vi "魔法攻击.vi"() -> ()   [LabVIEW 2018]
panel:
  out "滑动杆":dbl(slide) scale=0.0..10.0
  out "布尔 2":bool
  out "布尔":bool
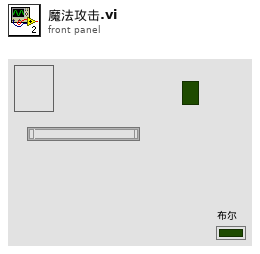
[diagram p1: front panel]
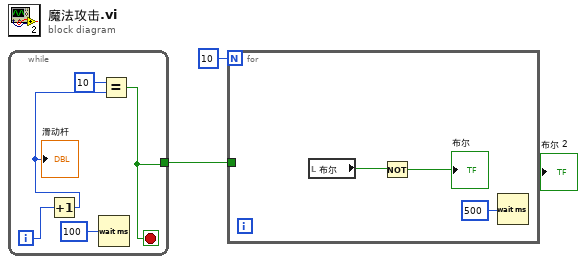
[diagram p0: block diagram]
diagram:
  n1 = while {
    tunnel: [w4] -> w1
    i -> [w7]
    stop <- w4 stop-if-true
    n2 = Increment(x=w7) -> (x+1=w6:i32)
    "滑动杆" <- w6
    n3 = Wait (ms)(milliseconds to wait=u32 100 ("等待时间（毫秒）")) -> ()  [unwired: 1 out]
    n4 = Equal?(x=10, y=w6) -> (x = y?=w4:bool)
  }
  n5 = for {
    N: 10 -> [_]
    tunnel: w1 -> [_]
    n6 = local read "布尔"() -> (w10:bool)
    n7 = Not(x=w10) -> (.not. x?=→"布尔":bool)
    n8 = Wait (ms)(milliseconds to wait=u32 500 ("毫秒计时值")) -> ()  [unwired: 1 out]
  }
